vi "CIMAQ Overlay Lines Big.vi"(6 "Overlay Thickness":i32(slide)=5 scale=0.0..20.0, 7 "Color":u32(colorbox)=16711680, 8 "error in (no error)":errorcluster, 9 "Point 2":cluster{"X":i32, "Y":i32}, 10 "Point 1":cluster{"X":i32, "Y":i32}, 11 "Image In":T1) -> (0 "error out":errorcluster, 3 "Image Out":T1)   [LabVIEW 2014]
uses:
  <vilib>/vision/Image Controls.llb/IMAQ Image.ctl
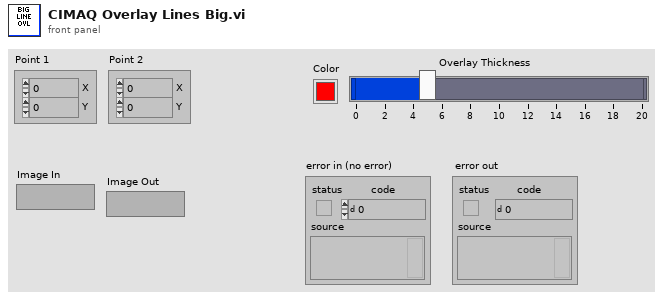
[diagram p1: front panel]
types:
  T1 = typedef "IMAQ Image.ctl" = refnum<image>
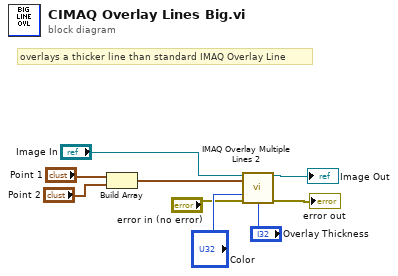
[diagram p0: block diagram]
diagram:
  # "overlays a thicker line than standard IMAQ Overlay Line"
  n1 = Build Array("Point 1", "Point 2") -> (w2:cluster{"X":i32, "Y":i32}[])
  n2 = call "IMAQ Overlay Multiple Lines 2"("Image"="Image In", "Line End Points"=w2, "Color"="Color", "error in (no error)"="error in (no error)", "Width"="Overlay Thickness") -> ("Image Out"=→"Image Out":T1, "error out"=→"error out":errorcluster)  [unwired: 9 in]
